vi "Data Analyisis Top Stack.vi"(2 "State Stack (in)":T1[](array[typedef])) -> (0 "State Stack (out)":T1[](array[typedef]), 1 "State (out)":T1=enum."Panel Monitoring")   [LabVIEW 2016]
uses:
  Data Analysis state.ctl
panel:
  # "Top Stack\nVER 1.0 AAM 10th April 2002\n\nThis VI removes the top element of the state stack \nand returns the remaining elements in the stack"
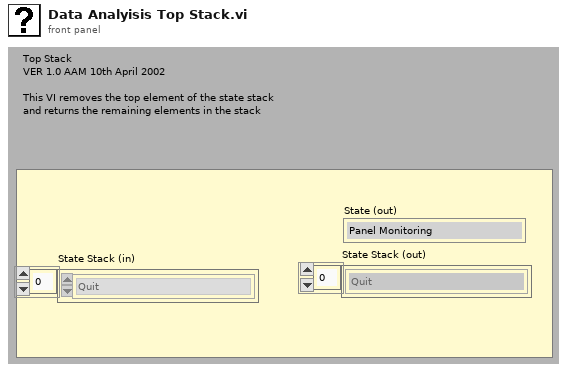
[diagram p1: front panel]
types:
  T1 = typedef "Data Analysis state.ctl" = enum16{"Quit", "Cycle Channels", "Generate Plot", "Analyse Data", "Save Image", "Polynomial Fit", "Open_Create Excel", "Excel find free A cell", "Panel Monitoring", "Save to Excel", "Initialize", "Extract Data", "Display Data", "Calculate Sinusoidal Gains", "Make Transient Fits & Equations", "Calculate Latency Fits", "Calculate Transient Ga 1 Gain", "Calculate Transient Ga 2 Gain", "Calculate Transient Gv Gain", "Stop", "Calculate Latency", "Calculate Exponential", "Calculate Mean", "Calculate Head Impulse", "Update controls and variables"}
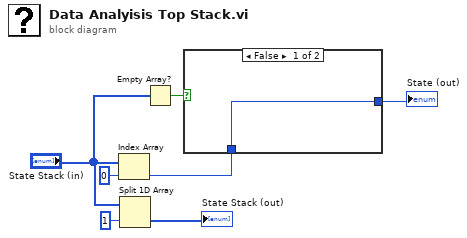
[diagram p0: block diagram]
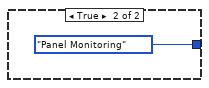
[diagram p2: hidden frame]
diagram:
  n1 = Index Array(array="State Stack (in)", index=0) -> (element=w3:T1)
  n2 = Split 1D Array(array="State Stack (in)", index=1) -> (second subarray=→"State Stack (out)":T1[])  [unwired: 1 out]
  n3 = Empty Array?(array="State Stack (in)") -> (empty?=w2:bool)
  n4 = case shown="False" w2 {
    tunnel: [w8 Data_Analysis_state."Panel Monitoring" ("State (out)")] -> w4
    tunnel: w3 -> [w8 _]
    frame False {
    }
    frame True {
    }
  }
  "State (out)" <- w4
